vi "set_params.vi"(8 "error in (no error)":errorcluster caption="entrée d'erreur (pas d'erreur)", 11 "OrthogonalMatchingPursuitCV.lvclass 2":refnum<class "OrthogonalMatchingPursuitCV.lvclass">) -> (0 "error out":errorcluster caption="sortie d'erreur", 3 "OrthogonalMatchingPursuitCV.lvclass":refnum<class "OrthogonalMatchingPursuitCV.lvclass">)   [LabVIEW 2020, in "OrthogonalMatchingPursuitCV.lvclass"]
uses:
  OrthogonalMatchingPursuitCV.lvclass
  OrthogonalMatchingPursuitCV.lvclass/OrthogonalMatchingPursuitCV.ctl
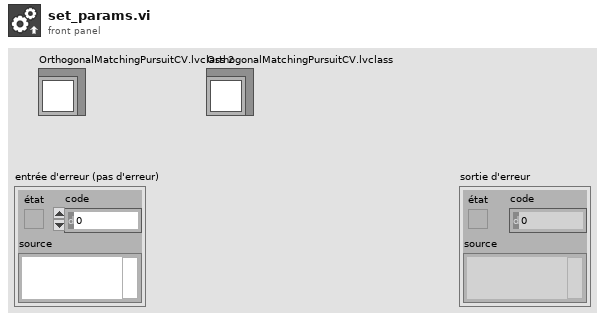
[diagram p1: front panel]
types:
  T1 = typedef "orthogonal_matching_pursuit_cv_params.ctl" = cluster{"copy":bool, "fit_intercept":bool, "normalize":bool, "max_iter":cluster{"max_iter_type":string, "max_iter_int":dbl}, "cv":dbl, "n_jobs":dbl, "verbose":cluster{"verbose_type":string, "verbose_bool":bool, "verbose_int":dbl}}
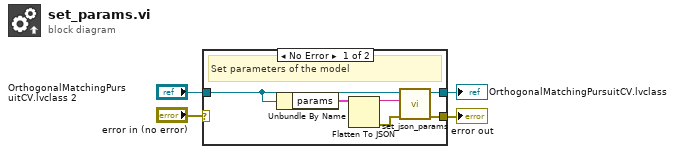
[diagram p0: block diagram]
diagram:
  n1 = case shown="No Error" "error in (no error)" {
    selector: "error in (no error)" -> [_ w12]
    tunnel: [w7 w12] -> w3
    tunnel: [w8 w11] -> w1
    tunnel: "OrthogonalMatchingPursuitCV.lvclass 2" -> [w5 w11]
    frame No Error {
      # "Set parameters of the model"
      n2 = Unbundle By Name(w5) -> ("params"=w10:T1)
      n3 = Flatten To JSON(anything=w10) -> (JSON string=w9:string, 11:w6:errorcluster)  [unwired: 2 in]
      n4 = call-dynamic "set_json_params.vi"("error in (no error)"=w6, "params"=w9, "Model en entrée"=w5) -> ("error out"=w7:errorcluster, "Model en sortie"=w8:refnum<class "OrthogonalMatchingPursuitCV.lvclass">)  [unwired: 7 in]
    }
    frame Error {
    }
  }
  "error out" <- w3
  "OrthogonalMatchingPursuitCV.lvclass" <- w1
